vi "Append Waveform.vi"(8 "Error":errorcluster, 9 "Waveform To Append":T1, 11 "(WavBuf)":refnum<class "(WavBuf).lvclass">) -> (0 "Error Out":errorcluster, 3 "(WavBuf) Out":refnum<class "(WavBuf).lvclass">)   [LabVIEW 2016, in "(WavBuf).lvclass"]
uses:
  (WavBuf).lvclass
  Universal Controls/Waveform_Data.ctl
  (WavBuf).lvclass/(WavBuf).ctl
  Support/Waveform_Read Write End Point Index.vi
  <vilib>/Waveform/WDTOps.llb/WDT Get Final Time Value DBL.vi
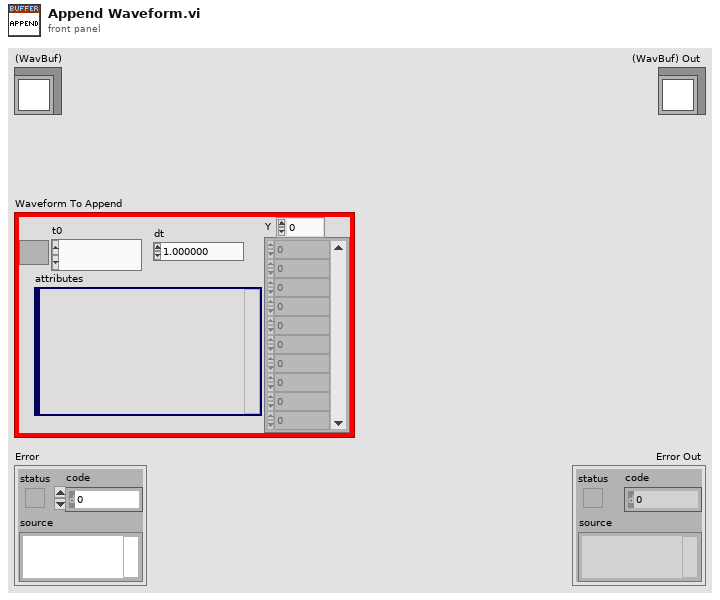
[diagram p1: front panel]
types:
  T1 = typedef "Waveform_Data.ctl" = waveform(dbl)
  T2 = typedef "Ref_DVR_Buffer.ctl" = refnum<data-value>
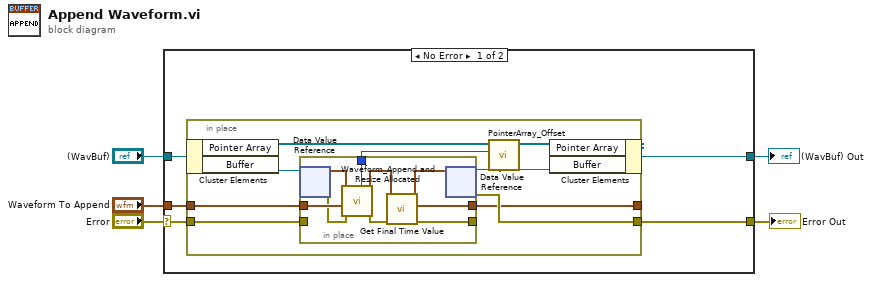
[diagram p0: block diagram]
diagram:
  n1 = case shown="No Error" "Error" {
    selector: "Error" -> [w8 w30]
    tunnel: [w6 w30] -> w4
    tunnel: [w10 w29] -> w2
    tunnel: "(WavBuf)" -> [w9 w29]
    tunnel: "Waveform To Append" -> [w7 _]
    frame No Error {
      n2 = in-place {
        in-place-border: w8 -> [w19]
        in-place-border: [w12] -> w6
        in-place-border: w7 -> [w18]
        in-place-border: [w11] -> _
        n3 = in-place-cluster #1(w9) -> ("Pointer Array"=w14:refnum<class "((Pointer)).lvclass">[], "Buffer"=w17:T2)
        n4 = in-place {
          in-place-border: w19 -> [_]
          in-place-border: [w21] -> _
          in-place-border: [w28] -> w15
          in-place-border: w18 -> [w26]
          in-place-border: [w20] -> w11
          n5 = in-place-dvr #2(w17) -> (w27:T1, w25:errorcluster)
          n6 = call "Waveform_Append and Resize Allocated.vi"("Error"=w25, "Append"=w26, "Waveform"=w27) -> ("Error Out"=w22:errorcluster, "Waveform Out"=w24:T1, "Offset Out"=w28:i32)  [unwired: 6 in]
          n7 = call-poly <vilib>:"Get Final Time Value.vi"("error in (no error)"=w22, "waveform in"=w24) -> ("error out"=w21:errorcluster, "tf"=w20:timestamp, "waveform out"=w23:waveform(dbl))  [unwired: 7 in]
          n8 = in-place-dvr #2(w23) -> (w16:T2, w12:errorcluster)
        }
        n9 = call "PointerArray_Offset.vi"("Buffer"=w16, "Total Starting Offset"=w15, "Pointer Array"=w14) -> ("Pointer Array Out"=w13:refnum<class "((Pointer)).lvclass">[])  [unwired: 8 in]
        n10 = in-place-cluster #1("Pointer Array"=w13, "Buffer"=w16) -> (w10:refnum<class "(WavBuf).lvclass">)
      }
    }
    frame Error {
    }
  }
  "Error Out" <- w4
  "(WavBuf) Out" <- w2
